vi "动态更新项目.vi"() -> ()   [LabVIEW 2012, in "Tree Tools.lvlib"]
uses:
  Tree Tools.lvlib
  Core Class/Tree Class/Tree Class.lvclass
  Core Class/Tree Tag Class/Tree Tag Class.lvclass
panel:
  out "Value":string[](array[string])
  out "Tag and Text":string[][](array[string])
  in  "Quit":bool
  in  "DI":T1
  in  "AD":T2
  in  "Device":string[](tree)
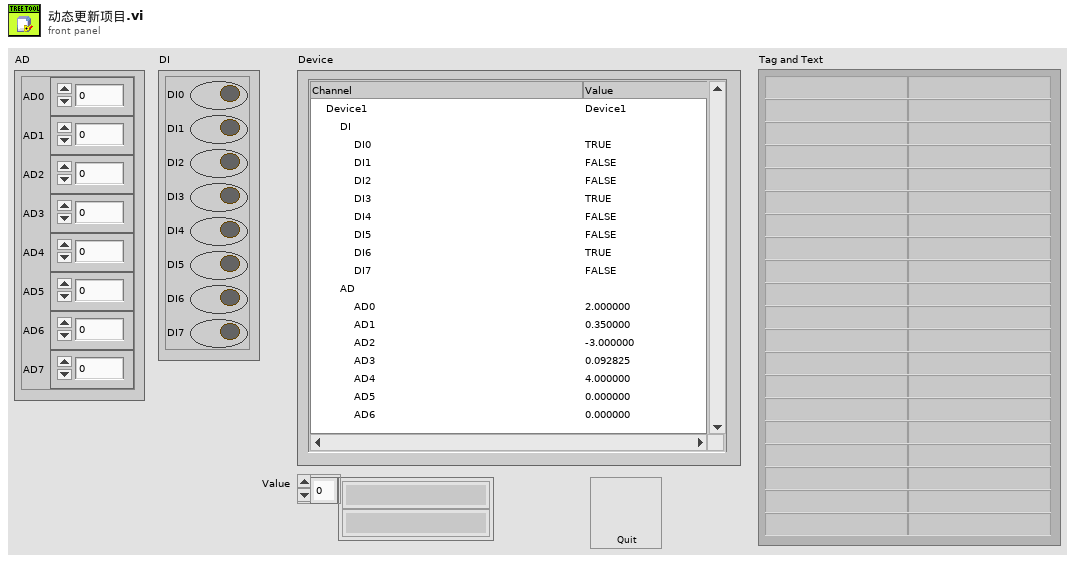
[diagram p1: front panel]
types:
  T1 = cluster{"DI0":bool, "DI1":bool, "DI2":bool, "DI3":bool, "DI4":bool, "DI5":bool, "DI6":bool, "DI7":bool}
  T2 = cluster{"AD0":dbl, "AD1":dbl, "AD2":dbl, "AD3":dbl, "AD4":dbl, "AD5":dbl, "AD6":dbl, "AD7":dbl}
  T3 = typedef "LVPoint32TypeDef.ctl" = cluster{"Horizontal":i32, "Vertical":i32}
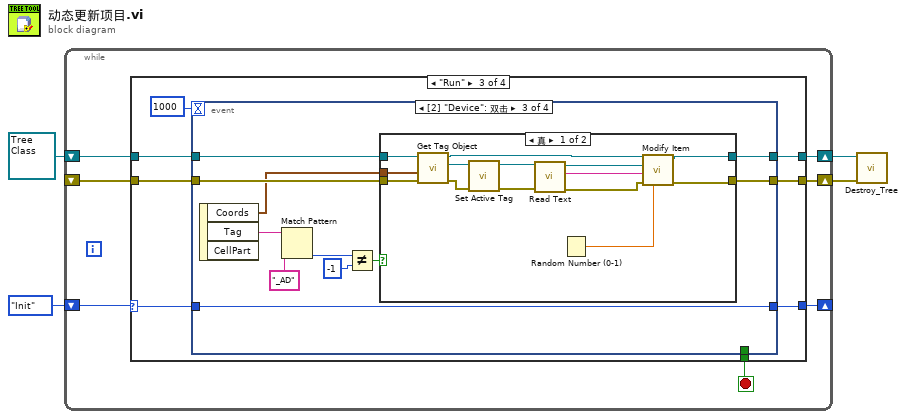
[diagram p0: block diagram]
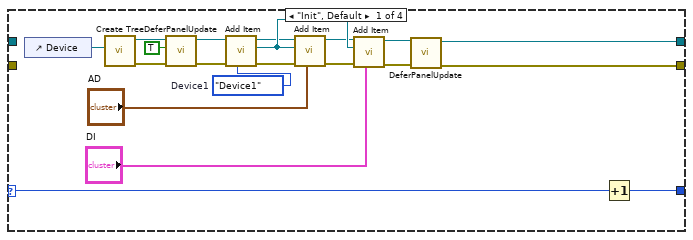
[diagram p2: hidden frame]
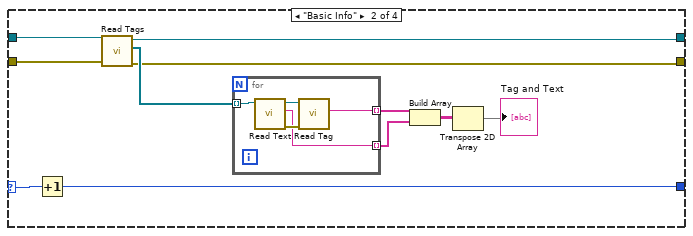
[diagram p3: hidden frame]
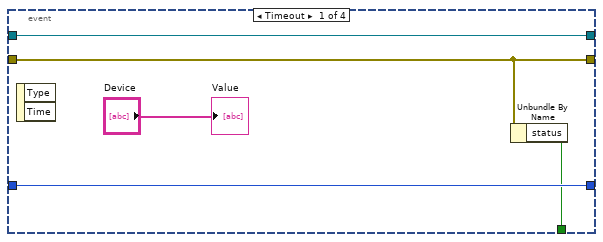
[diagram p4: hidden frame]
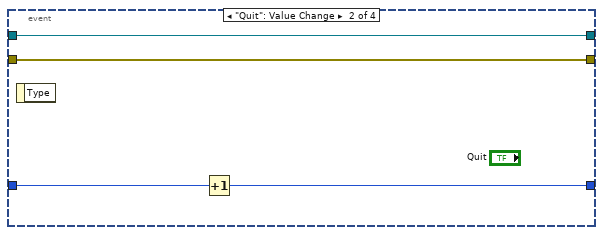
[diagram p5: hidden frame]
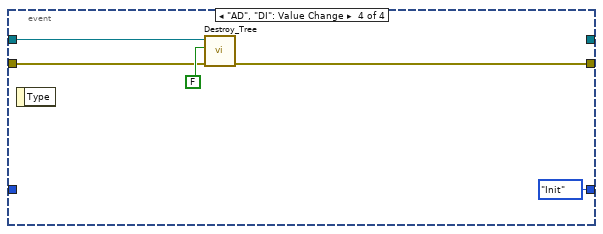
[diagram p7: hidden frame]
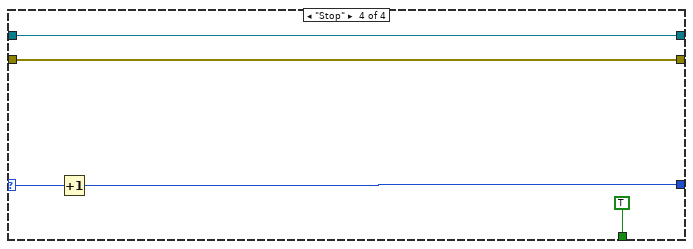
[diagram p8: hidden frame]
diagram:
  n1 = while {
    shift-right: [w7] -> w4
    shift-left: _ -> [w5]
    shift-right: [w8] -> w3
    shift-left: refnum<class "Tree Class.lvclass"> refnum ("Tree_LVOOP__lava_lib_tree_class out") -> [w6]
    shift-right: [w10] -> _
    shift-left: enum16{"Init", "Basic Info", "Run", "Stop"}."Init" -> [w11]
    stop <- w9 stop-if-true
    n2 = case shown="\"Run\"" w11 {
      selector: w11 -> [w31 w37 w51 w101]
      tunnel: [w30 w36 w50 w100] -> w10
      tunnel: [_ _ w48 TRUE] -> w9
      tunnel: [w13 w39 w54 w98] -> w8
      tunnel: [w12 w38 w52 w97] -> w7
      tunnel: w6 -> [_ w41 w55 w98]
      tunnel: w5 -> [_ w40 w53 w97]
      frame "Init", Default {
        w20 = enum16{"Device1", "Device2"}."Device1"  # Device1
        n3 = control-ref of="Device"() -> (w14:refnum<vi>)
        n4 = call "Create Tree.vi"("Tree Refnum"=w14) -> ("error out"=w16:errorcluster, "Tree_LVOOP out"=w15:refnum<class "Tree Class.lvclass">)  [unwired: 9 in]
        n5 = call-dynamic "DeferPanelUpdate.vi"("error in (no error)"=w16, "Defer? (F)"=TRUE, "Tree_LVOOP__lava_lib_tree_class in"=w15) -> ("error out"=w19:errorcluster, "Tree_LVOOP__lava_lib_tree_class out"=w18:refnum<class "Tree Class.lvclass">)  [unwired: 7 in]
        n6 = call-dynamic "Add Item.vi"("Data"=w20, "error in (no error)"=w19, "Tree_LVOOP in"=w18) -> ("error out"=w22:errorcluster, "Upmost Created Tag"=w27:refnum<class "Tree Tag Class.lvclass">, "Tree_LVOOP out"=w21:refnum<class "Tree Class.lvclass">)  [unwired: 6 in]
        n7 = call-dynamic "Add Item.vi"("Data"="AD", "error in (no error)"=w22, "Parent Tag"=w27, "Tree_LVOOP in"=w21) -> ("error out"=w24:errorcluster, "Tree_LVOOP out"=w25:refnum<class "Tree Class.lvclass">)  [unwired: 5 in, 1 out]
        n8 = call-dynamic "Add Item.vi"("Data"="DI", "error in (no error)"=w24, "Parent Tag"=w27, "Tree_LVOOP in"=w25) -> ("error out"=w29:errorcluster, "Tree_LVOOP out"=w28:refnum<class "Tree Class.lvclass">)  [unwired: 5 in, 1 out]
        n9 = call-dynamic "DeferPanelUpdate.vi"("error in (no error)"=w29, "Tree_LVOOP__lava_lib_tree_class in"=w28) -> ("error out"=w12:errorcluster, "Tree_LVOOP__lava_lib_tree_class out"=w13:refnum<class "Tree Class.lvclass">)  [unwired: 8 in]
        n10 = Increment(x=w31) -> (x+1=w30:enum16{"Init", "Basic Info", "Run", "Stop"})
      }
      frame "Basic Info" {
        n11 = Increment(x=w37) -> (x+1=w36:enum16{"Init", "Basic Info", "Run", "Stop"})
        n12 = call-dynamic "Read Tags.vi"("error in (no error)"=w40, "Tree_LVOOP__lava_lib_tree_class in"=w41) -> ("error out"=w38:errorcluster, "Tags"=w42:refnum<class "Tree Tag Class.lvclass">[], "Tree_LVOOP__lava_lib_tree_class out"=w39:refnum<class "Tree Class.lvclass">)  [unwired: 7 in]
        n13 = for {
          tunnel: [w45] -> w34 mode=indexing
          tunnel: [w44] -> w35 mode=indexing
          tunnel: w42 -> [w43] mode=indexing
          n14 = call-dynamic "Read Text.vi"("Tag_LVOOP.lvclass in"=w43) -> ("error out"=w46:errorcluster, "Text"=w45:string, "Tag_LVOOP.lvclass out"=w47:refnum<class "Tree Tag Class.lvclass">)  [unwired: 8 in]
          n15 = call-dynamic "Read Tag.vi"("error in (no error)"=w46, "Tag_LVOOP.lvclass in"=w47) -> ("Tag"=w44:string)  [unwired: 7 in, 2 out]
        }
        n16 = Build Array(w35, w34) -> (w33:string[][])
        n17 = Transpose 2D Array(2D array=w33) -> (transposed array=→"Tag and Text":string[][])
      }
      frame "Run" {
        n18 = event shown="[2] \"Device\": 双击" {
          selector: _ -> [_ _ _ _]
          dyn-events: _ -> [_ _ _ _]
          timeout: 1000 -> [_ _ _ _]
          tunnel: w55 -> [w60 w64 w74 w95]
          tunnel: [w60 w64 w72 _] -> w54
          tunnel: w53 -> [w58 w63 w73 w93]
          tunnel: [w58 w63 w71 w92] -> w52
          tunnel: [w59 w61 w75 enum16{"Init", "Basic Info", "Run", "Stop"}."Init"] -> w50
          tunnel: w51 -> [w59 w62 w75 _]
          tunnel: [w57 _ _ _] -> w48
          event Timeout {
            n19 = event-data() -> ()  [unwired: 1 in, 2 out]
            n20 = Unbundle By Name(w58) -> ("status"=w57:bool)
            "Value" <- "Device"
          }
          event "Quit": Value Change {
            n21 = event-data() -> ()  [unwired: 1 in, 1 out]
            n22 = Increment(x=w62) -> (x+1=w61:enum16{"Init", "Basic Info", "Run", "Stop"})
          }
          event "Device": Double Click {
            n23 = event-data() -> ("Coords"=w65:T3, "Tag"=w66:string)  [unwired: 1 in, 1 out]
            n24 = Match Pattern(string=w66, regular expression="_AD" ("替换字符串(\"\")")) -> (offset past match=w69:i32)  [unwired: 1 in, 3 out]
            n25 = Not Equal?(x=w69, y=-1) -> (x != y?=w67:bool)
            n26 = case shown="真" w67 {
              tunnel: w74 -> [w89 w91]
              tunnel: w73 -> [w88 w90]
              tunnel: [w81 w91] -> w72
              tunnel: w65 -> [w87 _]
              tunnel: [w77 w90] -> w71
              frame True {
                n27 = call-dynamic "Get Tag Object.vi"("error in (no error)"=w88, "Coords (if tag empty)"=w87, "Tree_LVOOP in"=w89) -> ("error out"=w85:errorcluster, "Tag"=w86:refnum<class "Tree Tag Class.lvclass">, "Tree_LVOOP out"=w82:refnum<class "Tree Class.lvclass">)  [unwired: 5 in, 1 out]
                n28 = call-dynamic "Set Active Tag.vi"("error in (no error)"=w85, "Tag_LVOOP in"=w86) -> ("error out"=w83:errorcluster, "Tag_LVOOP out"=w84:refnum<class "Tree Tag Class.lvclass">)  [unwired: 8 in]
                n29 = call-dynamic "Read Text.vi"("error in (no error)"=w83, "Tag_LVOOP.lvclass in"=w84) -> ("error out"=w76:errorcluster, "Text"=w79:string, "Tag_LVOOP.lvclass out"=w80:refnum<class "Tree Tag Class.lvclass">)  [unwired: 7 in]
                n30 = Random Number (0-1) ("kkkkk")() -> (number: 0 to 1=w78:dbl)
                n31 = call-dynamic "Modify Item.vi"("Data"=w78, "error in (no error)"=w76, "Text"=w79, "Tag"=w80, "Tree_LVOOP in"=w82) -> ("error out"=w77:errorcluster, "Tree_LVOOP out"=w81:refnum<class "Tree Class.lvclass">)  [unwired: 4 in, 1 out]
              }
              frame False {
              }
            }
          }
          event "AD", "DI": Value Change {
            n32 = event-data() -> ()  [unwired: 1 in, 1 out]
            n33 = call-dynamic "Destroy_Tree.vi"("error in (no error)"=w93, "Delete Tree Items? (F)"=FALSE, "Tree_LVOOP in"=w95) -> ("error out"=w92:errorcluster)  [unwired: 8 in]
          }
        }
      }
      frame "Stop" {
        n34 = Increment(x=w101) -> (x+1=w100:enum16{"Init", "Basic Info", "Run", "Stop"})
      }
    }
  }
  n35 = call-dynamic "Destroy_Tree.vi"("error in (no error)"=w4, "Tree_LVOOP in"=w3) -> ()  [unwired: 9 in, 1 out]
